vi "9350_UI.vi"(8 "error in (no error)":errorcluster, 11 "Node Ptr":T1 format="%.0x") -> (0 "error out":errorcluster)   [LabVIEW 2019, in "Modules.lvlib" / "9350.lvclass"]
uses:
  9350.lvclass
  <vilib>/NI VeriStand/Custom Device API/Custom Device Item Ref.ctl
  RSI Module/SubPanel Command.ctl
  <vilib>/NI VeriStand/Custom Device API/Custom Device API.lvlib
  RSI Module/RSI Module.lvclass
panel:
  in  "SubPanel Event":refnum<user-event>
  # "This module provides read-only support for NI-9350 channels.\n\nUse the Functional Safety Editor to create and compile a safety program for your module and LabVIEW to deploy the resulting .bin file. The safety program must be set to automatically start."
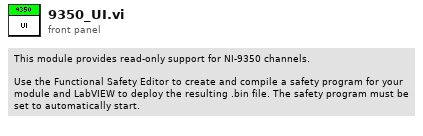
[diagram p1: front panel]
types:
  T1 = typedef "Custom Device API.lvlib/Custom Device Item Ref.ctl" = u64
  T2 = typedef "Modules.lvlib/RSI Module.lvclass/SubPanel Command.ctl" = enum16{"Stop"}
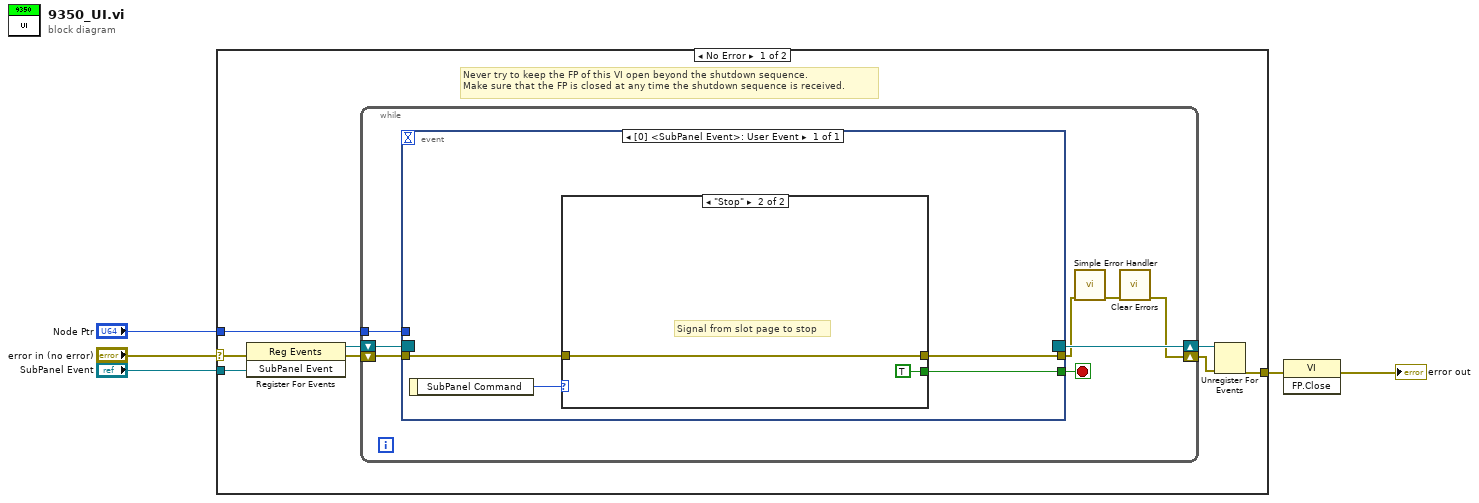
[diagram p0: block diagram]
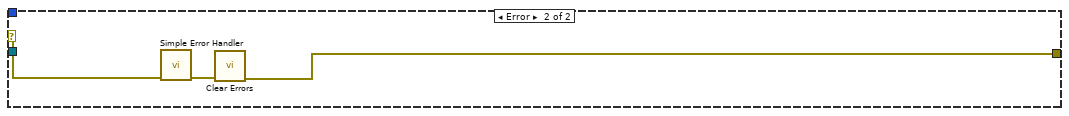
[diagram p3: hidden frame]
diagram:
  n1 = case shown="No Error" "error in (no error)" {
    selector: "error in (no error)" -> [w7 w31]
    tunnel: [w11 w29] -> w5
    tunnel: "Node Ptr" -> [w8 _]
    tunnel: "SubPanel Event" -> [w6 _]
    frame No Error {
      # "Never try to keep the FP of this VI open beyond the shutdown sequence.\nMake sure that the FP is closed at any time the shutdown sequence is received."
      n2 = register-events(error in=w7, w6) -> (reference out=w9:refnum<event-registration>, error out=w10:errorcluster)  [unwired: 1 in]
      n3 = while {
        tunnel: w8 -> [w17]
        shift-right: [w14] -> w12
        shift-left: w10 -> [w20]
        shift-right: [w21] -> w13
        shift-left: w9 -> [w19]
        stop <- w18 stop-if-true
        n4 = event shown="[0] <SubPanel Event>: User Event" {
          selector: w19 -> [_]
          dyn-events: [_] -> w21
          timeout: _ -> [_]
          tunnel: w20 -> [w24]
          tunnel: [w23] -> w18
          tunnel: [w22] -> w16
          tunnel: w17 -> [_]
          event User Event {
            n5 = event-data() -> ("SubPanel Command"=w25:T2)  [unwired: 1 out]
            n6 = case shown="\"Stop\"" w25 {
              tunnel: w24 -> [w26 w27]
              tunnel: [w26 w27] -> w22
              tunnel: [_ TRUE] -> w23
              frame Default {
              }
              frame "Stop" {
                # "Signal from slot page to stop"
              }
            }
          }
        }
        n7 = call <vilib>:"Simple Error Handler.vi"("error in (no error)"=w16) -> ("error out"=w15:errorcluster)  [unwired: 1 in, 7 out]
        n8 = call <vilib>:"Clear Errors.vi"("error in (no error)"=w15) -> ("error out"=w14:errorcluster)  [unwired: 1 in, 5 out]
      }
      n9 = Unregister For Events(event registration refnum=w13, error in=w12) -> (error out=w11:errorcluster)
    }
    frame Error {
      n10 = call <vilib>:"Simple Error Handler.vi"("error in (no error)"=w31) -> ("error out"=w30:errorcluster)  [unwired: 1 in, 7 out]
      n11 = call <vilib>:"Clear Errors.vi"("error in (no error)"=w30) -> ("error out"=w29:errorcluster)  [unwired: 1 in, 5 out]
    }
  }
  n12 = invoke class="VI" method="FP.Close"(error in=w5) -> (error out=→"error out":errorcluster)  [unwired: 2 in, 2 out]
